vi "Get_Devices.vi"(8 "error in (no error)":errorcluster) -> (0 "error out":errorcluster, 2 "devices":T1(array[cluster]))   [LabVIEW 2019, in "Kinova MICO² USB.lvlib"]
uses:
  <vilib>/Utility/error.llb/Error Cluster From Error Code.vi
  <vilib>/ErrorRing/Error Ring.xnode
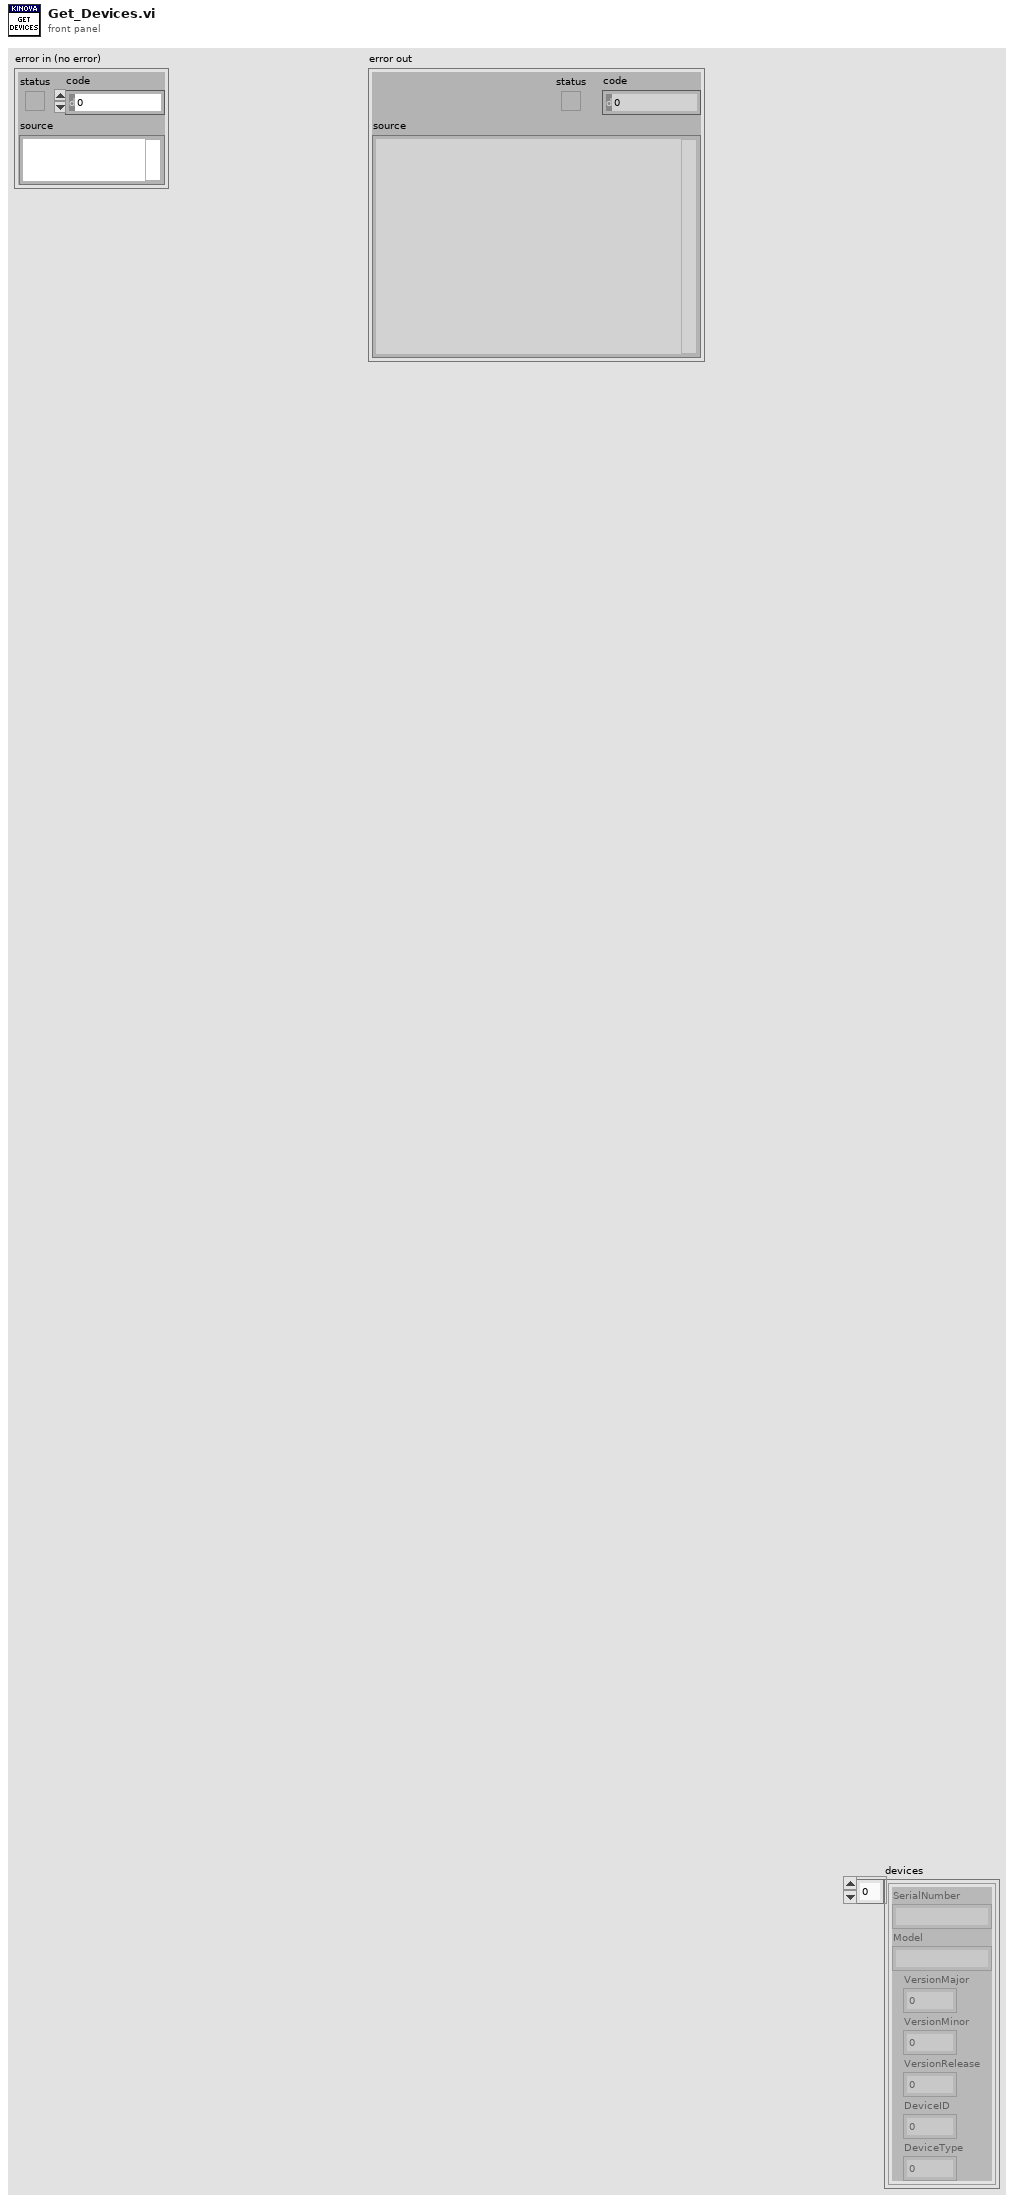
[diagram p1: front panel]
types:
  T1 = cluster{"SerialNumber":string, "Model":string, "VersionMajor":i32, "VersionMinor":i32, "VersionRelease":i32, "DeviceID":i32, "DeviceType":i32}[]
  T2 = cluster{"SerialNumber":string, "Model":string, "VersionMajor":i32, "VersionMinor":i32, "VersionRelease":i32, "DeviceID":i32, "DeviceType":i32}
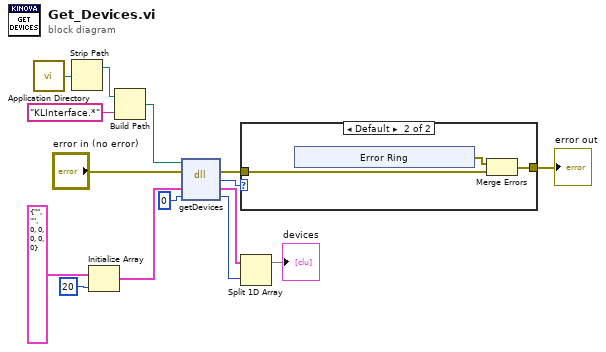
[diagram p0: block diagram]
diagram:
  n1 = call <vilib>:"Application Directory.vi"() -> ("Application Directory"=w1:path)
  n2 = Strip Path(path=w1) -> (stripped path=w13:path)  [unwired: 1 out]
  n3 = Initialize Array(T2 {"SerialNumber"="", "Model"="", "VersionMajor"=0, "VersionMinor"=0, "VersionRelease"=0, "DeviceID"=0, "DeviceType"=0} ("Kinova Device"), 20 ("dimension size")) -> (w8:T1)
  n4 = Build Path(base path=w13, name or relative path="KLInterface.*") -> (appended path=w2:path)
  n5 = dll-call lib="C:/Users/mcjssdcc/source/repos/Kinova Labview Interface/Debug/KLInterface.dll" fn="getDevices"(path in=w2, error in="error in (no error)", "devices"=w8, "devicecount"=0) -> (error out=w12:errorcluster, "return type"=w10:i32, "devices"=w5:T1, "devicecount"=w6:i32)  [unwired: 1 in, 1 out]
  n6 = case shown="Default" w10 {
    tunnel: [w16 w18] -> w11
    tunnel: w12 -> [w16 w17]
    frame 1 {
    }
    frame Default {
      n7 = xnode "Error Ring"() -> ("error out"=w19:errorcluster)
      n8 = Merge Errors(w19, w17) -> (w18:errorcluster)
    }
  }
  "error out" <- w11
  n9 = Split 1D Array(array=w5, index=w6) -> (first subarray=→"devices":T1)  [unwired: 1 out]
